vi "Write Strict refs box.vi"(8 "error in (no error)":errorcluster, 10 "Strict refs box":T1, 11 "BLE context in":refnum<class "BLE context.lvclass">) -> (0 "error out":errorcluster, 3 "BLE context out":refnum<class "BLE context.lvclass">)   [LabVIEW 2015, in "BLE context.lvclass"]
uses:
  BLE context.lvclass
  ctrls/RefsBox.ctl
  BLE context.lvclass/BLE context.ctl
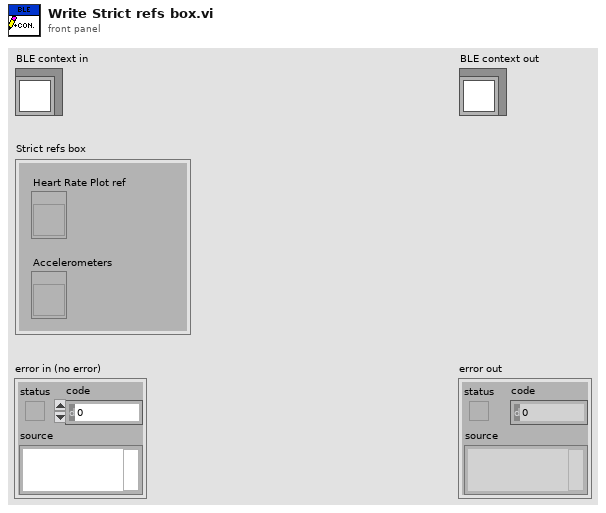
[diagram p1: front panel]
types:
  T1 = typedef "RefsBox.ctl" = cluster{"Heart Rate Plot ref":refnum<vi>, "Accelerometers":refnum<vi>}
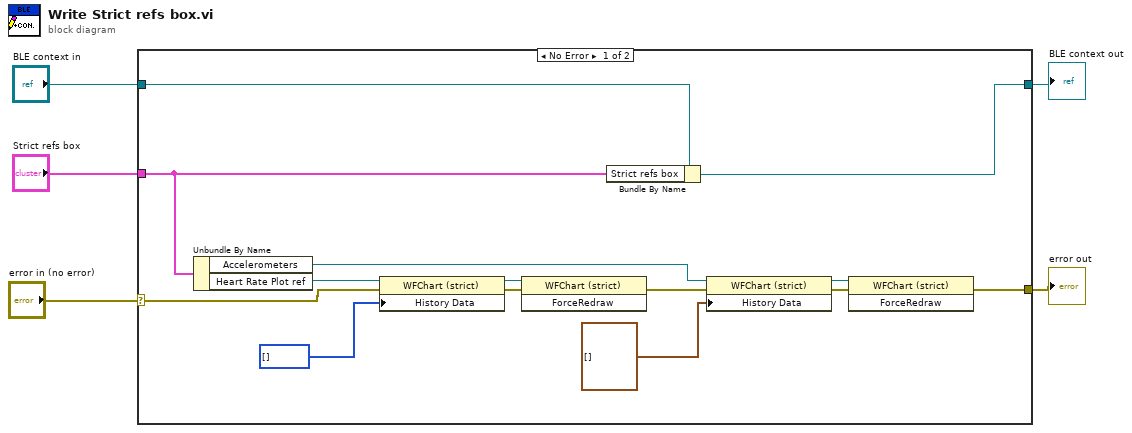
[diagram p0: block diagram]
diagram:
  n1 = case shown="No Error" "error in (no error)" {
    selector: "error in (no error)" -> [w12 w20]
    tunnel: [w6 w20] -> w4
    tunnel: [w18 w21] -> w2
    tunnel: "BLE context in" -> [w19 w21]
    tunnel: "Strict refs box" -> [w17 _]
    frame No Error {
      n2 = Unbundle By Name(w17) -> ("Accelerometers"=w8:refnum<vi>, "Heart Rate Plot ref"=w15:refnum<vi>)
      n3 = property on="Property Node" class="WFChart (strict)"(reference=w15, error in=w12, "History Data"=u32[] []) -> (reference out=w14:refnum<vi>, error out=w16:errorcluster)
      n4 = invoke on="Invoke Node" class="WFChart (strict)" method="ForceRedraw"(reference=w14, error in=w16) -> (error out=w9:errorcluster)  [unwired: 1 in, 2 out]
      n5 = Bundle By Name(cluster=w19, "Strict refs box"=w17) -> (w18:refnum<class "BLE context.lvclass">)
      n6 = property on="Property Node" class="WFChart (strict)"(reference=w8, error in=w9, "History Data"=cluster{dbl, dbl, dbl}[] []) -> (reference out=w11:refnum<vi>, error out=w10:errorcluster)
      n7 = invoke on="Invoke Node" class="WFChart (strict)" method="ForceRedraw"(reference=w11, error in=w10) -> (error out=w6:errorcluster)  [unwired: 1 in, 2 out]
    }
    frame Error {
    }
  }
  "error out" <- w4
  "BLE context out" <- w2
